vi "TC GUI v2.vi"() -> ()   [LabVIEW 2016]
uses:
  <vilib>/Utility/file.llb/Write Delimited Spreadsheet (string).vi
  <vilib>/Utility/file.llb/Write Delimited Spreadsheet (DBL).vi
panel:
  out "Fiber Coupler":dbl
  out "Waveform Chart":T1(graph)
  out "TC 19":dbl
  out "TC 18":dbl
  out "TC 17":dbl
  out "TC 16":dbl
  out "TC 15":dbl
  out "TC 14\n(Side of Ti Plate)":dbl
  out "TC 13 \n(Laser Magnet TC)":dbl
  out "TC 12 \n(Center \nThreaded on \nFixture)":dbl
  out "TC 11 \n(Comp Magnet TC)":dbl
  out "Camer Right\n Angle Mirror":dbl
  out "Optics":dbl
  out "Camera":dbl
  out "Free Floating":dbl
  out "Cover Slide \nModule":dbl
  out "Bottom\n Downtube":dbl
  out "Aluminum \nCooling Block":dbl
  out "Copper Plate":dbl
  out "Nozzle":dbl
  in  "base path":path=path "C:/Users/Mark/Desktop/BeadScan"
  in  "stop":bool
  # "See TC Drawing for TC's 15 through 19"
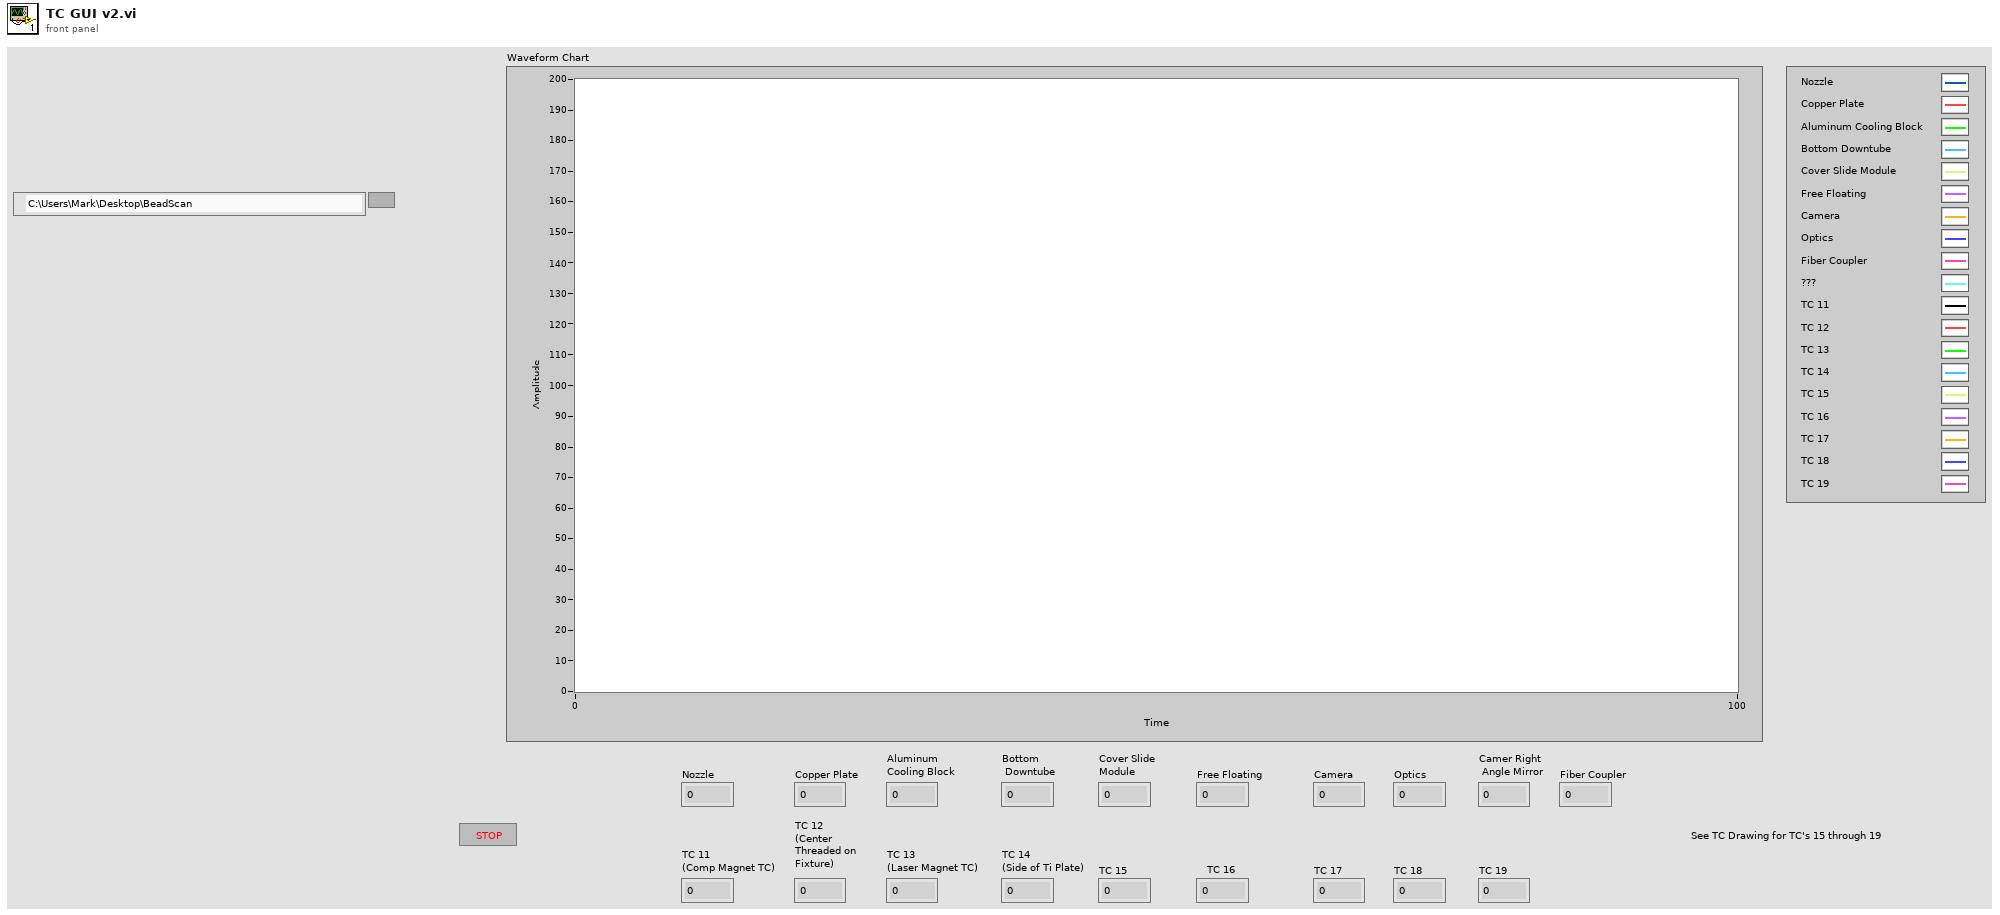
[diagram p1: front panel]
types:
  T1 = cluster{"Array of Double[0]":dbl, "Array of Double[1]":dbl, "Array of Double[2]":dbl, "Array of Double[3]":dbl, "Array of Double[4]":dbl, "Array of Double[5]":dbl, "Array of Double[6]":dbl, "Array of Double[7]":dbl, "Array of Double[8]":dbl}
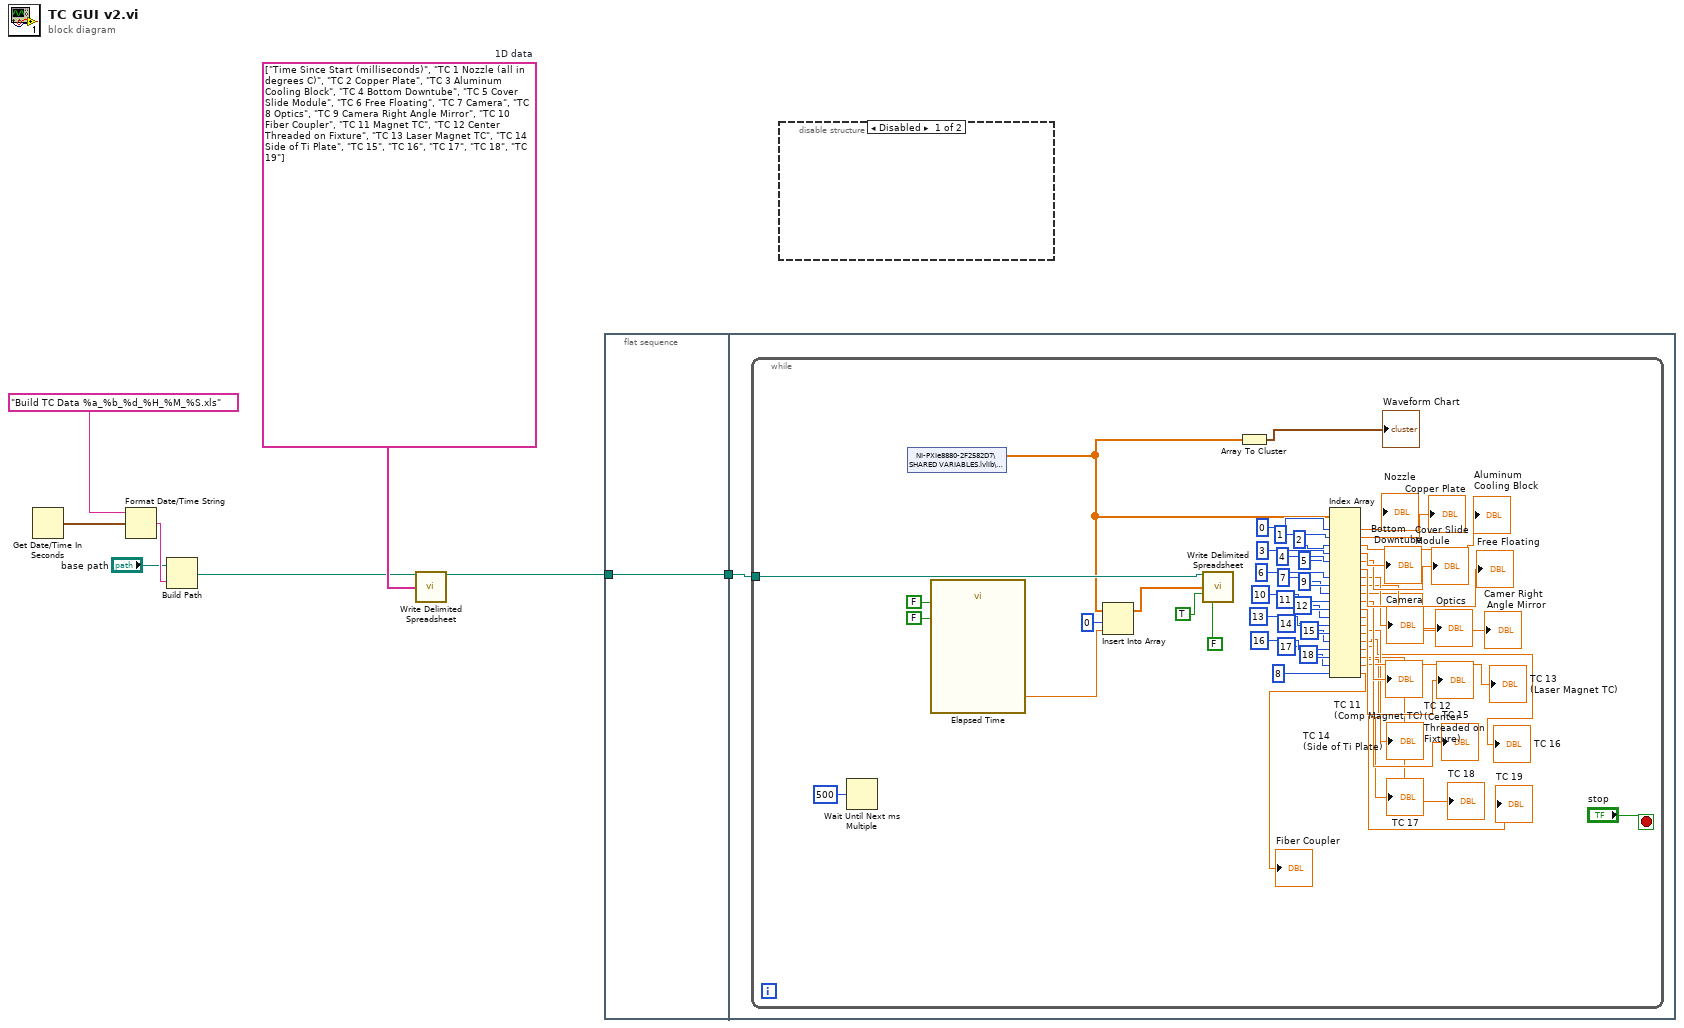
[diagram p0: block diagram]
diagram:
  w5 = string[] ["Time Since Start (milliseconds)", "TC 1 Nozzle (all in degrees C)", "TC 2 Copper Plate", "TC 3 Aluminum Cooling Block", "TC 4 Bottom Downtube", "TC 5 Cover Slide Module", "TC 6 Free Floating", "TC 7 Camera", "TC 8 Optics", "TC 9 Camera Right Angle Mirror", "TC 10 Fiber Coupler", "TC 11 Magnet TC", "TC 12 Center Threaded on Fixture", "TC 13 Laser Magnet TC", "TC 14 Side of Ti Plate", "TC 15", "TC 16", "TC 17", "TC 18", "TC 19"]  # 1D data
  n1 = Get Date/Time In Seconds() -> (seconds since 1Jan1904=w8:timestamp)
  n2 = Format Date/Time String(time format string (%c)="Build TC Data %a_%b_%d_%H_%M_%S.xls", seconds (now)=w8) -> (date/time string=w6:string)  [unwired: 1 in]
  n3 = Build Path(base path="base path", name or relative path=w6) -> (appended path=w4:path)
  n4 = call-poly <vilib>:"Write Delimited Spreadsheet.vi"("file path (dialog if empty)"=w4, "1D data"=w5) -> ("new file path (Not A Path if cancelled)"=w2:path)  [unwired: 12 in, 1 out]
  n5 = flat-sequence {
    tunnel: w2 -> [w9]
    tunnel: [w9] -> w1
    tunnel: w1 -> [w10]
    frame #0 {
    }
    frame #1 {
      n6 = while {
        tunnel: w10 -> [w58]
        stop <- "stop" stop-if-true
        n7 = Wait Until Next ms Multiple(millisecond multiple=u32 500) -> ()  [unwired: 1 out]
        n8 = shared-variable "NI-PXIe8880-2F2582D7\\SHARED VARIABLES.lvlib\\TC's Array"() -> (w14:dbl[])  [unwired: 1 in, 1 out]
        n9 = call "Elapsed Time"("Reset"=FALSE, "Auto Reset"=FALSE) -> ("Elapsed Time (s)"=w53:dbl)  [unwired: 10 in, 7 out]
        n10 = Insert Into Array(array=w14, index=0, new element=w53) -> (w54:dbl[])
        n11 = call-poly <vilib>:"Write Delimited Spreadsheet.vi"("file path (dialog if empty)"=w58, "1D data"=w54, "append to file? (new file:F)"=TRUE, "transpose? (no:F)"=FALSE) -> ()  [unwired: 10 in, 2 out]
        n12 = Array To Cluster(array=w14) -> (cluster=→"Waveform Chart":T1)
        n13 = Index Array(array=w14, index #1=0 ("index"), index #2=1 ("index"), index #3=2 ("index"), index #4=3 ("index"), index #5=4 ("index"), index #6=5 ("index"), index #7=6 ("index"), index #8=7 ("index"), index #9=9 ("index"), index #10=10 ("index"), index #11=11 ("index"), index #12=12 ("index"), index #13=13 ("index"), index #14=14 ("index"), index #15=15 ("index"), index #16=16 ("index"), index #17=17 ("index"), index #18=18 ("index"), index #19=8 ("index")) -> (element #1=→"Nozzle":dbl, element #2=→"Copper Plate":dbl, element #3=→"Aluminum \nCooling Block":dbl, element #4=→"Bottom\n Downtube":dbl, element #5=→"Cover Slide \nModule":dbl, element #6=→"Free Floating":dbl, element #7=→"Camera":dbl, element #8=→"Optics":dbl, element #9=→"Camer Right\n Angle Mirror":dbl, element #10=→"TC 11 \n(Comp Magnet TC)":dbl, element #11=→"TC 12 \n(Center \nThreaded on \nFixture)":dbl, element #12=→"TC 13 \n(Laser Magnet TC)":dbl, element #13=→"TC 14\n(Side of Ti Plate)":dbl, element #14=→"TC 15":dbl, element #15=→"TC 16":dbl, element #16=→"TC 17":dbl, element #17=→"TC 18":dbl, element #18=→"TC 19":dbl, element #19=→"Fiber Coupler":dbl)
      }
    }
  }
  n14 = disable-structure shown="Disabled" {
    frame Disabled {
    }
    frame Enabled {
    }
  }
